vi "HTML Report Get Font Formatting.vi"(7 "String In":string="<FONT FACE=\"Arial\" COLOR=\"#FF00FF\">\n<I><STRIKE><U><B>") -> (0 "font settings":T1, 1 "Text Options":T2, 2 "Color Box":u32(colorbox), 3 "Output Element":cluster{"red":u8, "green":u8, "blue":u8})   [LabVIEW 2020, in "NI_ReportGenerationCore.lvlib"]
uses:
  <vilib>/Utility/NIReport.llb/NI_ReportGenerationCore.lvlib
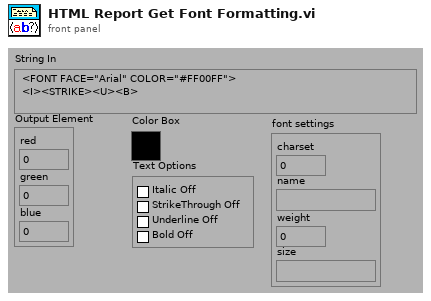
[diagram p1: front panel]
types:
  T1 = cluster{"charset":i16, "name":string, "weight":i16, "size":string}
  T2 = cluster{"Italic":bool, "StrikeThrough":bool, "Underline":bool, "Bold":bool}
  T3 = cluster{"Charset":i16, "name":string, "Weight":i16, "size":string}
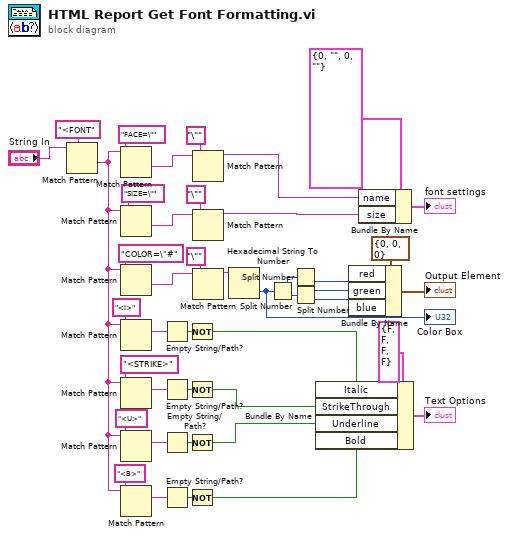
[diagram p0: block diagram]
diagram:
  n1 = Match Pattern(string="String In", regular expression="<FONT") -> (after substring=w10:string)  [unwired: 4 out]
  n2 = Match Pattern(string=w10, regular expression="FACE=\"") -> (after substring=w36:string)  [unwired: 4 out]
  n3 = Match Pattern(string=w10, regular expression="SIZE=\"") -> (after substring=w13:string)  [unwired: 4 out]
  n4 = Match Pattern(string=w10, regular expression="COLOR=\"#") -> (after substring=w39:string)  [unwired: 4 out]
  n5 = Match Pattern(string=w10, regular expression="<I>") -> (match substring=w31:string)  [unwired: 4 out]
  n6 = Match Pattern(string=w10, regular expression="<STRIKE>") -> (match substring=w30:string)  [unwired: 4 out]
  n7 = Match Pattern(string=w10, regular expression="<U>") -> (match substring=w29:string)  [unwired: 4 out]
  n8 = Match Pattern(string=w10, regular expression="<B>") -> (match substring=w28:string)  [unwired: 4 out]
  n9 = Empty String/Path?(string/path=w31) -> (empty?=w27:bool)
  n10 = Empty String/Path?(string/path=w30) -> (empty?=w26:bool)
  n11 = Empty String/Path?(string/path=w29) -> (empty?=w25:bool)
  n12 = Empty String/Path?(string/path=w28) -> (empty?=w24:bool)
  n13 = Not(x=w27) -> (.not. x?=w4:bool)
  n14 = Not(x=w26) -> (.not. x?=w3:bool)
  n15 = Not(x=w25) -> (.not. x?=w2:bool)
  n16 = Not(x=w24) -> (.not. x?=w5:bool)
  n17 = Match Pattern(string=w36, regular expression="\"") -> (before substring=w15:string)  [unwired: 4 out]
  n18 = Match Pattern(string=w13, regular expression="\"") -> (before substring=w9:string)  [unwired: 4 out]
  n19 = Match Pattern(string=w39, regular expression="\"") -> (before substring=w23:string)  [unwired: 4 out]
  n20 = Hexadecimal String To Number(string=w23) -> (number=w17:u32)  [unwired: 3 out]
  "Color Box" <- w17
  n21 = Split Number(x=w17) -> (hi(x)=w21:u16, lo(x)=w20:u16)
  n22 = Split Number(x=w21) -> (lo(x)=w18:u8)  [unwired: 1 out]
  n23 = Split Number(x=w20) -> (hi(x)=w19:u8, lo(x)=w16:u8)
  n24 = Bundle By Name(cluster=T2 {"Italic"=FALSE, "StrikeThrough"=FALSE, "Underline"=FALSE, "Bold"=FALSE} ("Text Options"), "Italic"=w4, "StrikeThrough"=w3, "Underline"=w2, "Bold"=w5) -> (→"Text Options":T2)
  n25 = Bundle By Name(cluster=cluster{"red":u8, "green":u8, "blue":u8} {"red"=0, "green"=0, "blue"=0} ("Output Element"), "red"=w18, "green"=w19, "blue"=w16) -> (→"Output Element":cluster{"red":u8, "green":u8, "blue":u8})
  n26 = Bundle By Name(cluster=T3 {"Charset"=0, "name"="", "Weight"=0, "size"=""}, "name"=w15, "size"=w9) -> (→"font settings":T3)
